vi "dfd_Set Bank Coef Infos.vi"(7 "type":T7, 8 "error in (no error)":errorcluster, 9 "gain":dbl, 10 "coefficients":dbl[](array[numeric]), 11 "bank in":T1={"mBank_Filters"=[], " mBank_#Bands"=2, "mBank_ProcMethod"=enum."General", "mBank_Coeffs"=[], "mBank_Gain"=1.0, "mBank_Type"=0} {"mBank_Type" items=["Uniform", "Non-Uniform"]; "mBank_Filters"."mMRate_SumWl" min=1 max=32 step=1; "mBank_Filters"."mMRate_InputIwl" min=1 max=32 step=1; "mBank_Filters"."mMRate_GainWl" min=1 max=32 step=1; "mBank_Filters"."mMRate_OutputWl" min=1 max=32 step=1; "mBank_Filters"."mMRate_InputWl" min=1 max=32 step=1; "mBank_Filters"."mMRate_CoefWl" min=1 max=32 step=1; "mBank_Filters"."mMRate_Mode" items=["Default"=-1, "No Rate Change"=0, "Interpolation"=1, "Decimation"=2, "Interpolated"=3, "Rational"=4]}) -> (0 "error out":errorcluster, 3 "bank out":T1={"mBank_Filters"=[], " mBank_#Bands"=2, "mBank_ProcMethod"=enum."General", "mBank_Coeffs"=[], "mBank_Gain"=1.0, "mBank_Type"=0} {"mBank_Type" items=["Uniform", "Non-Uniform"]; "mBank_Filters"."mMRate_SumWl" min=1 max=32 step=1; "mBank_Filters"."mMRate_InputIwl" min=1 max=32 step=1; "mBank_Filters"."mMRate_GainWl" min=1 max=32 step=1; "mBank_Filters"."mMRate_OutputWl" min=1 max=32 step=1; "mBank_Filters"."mMRate_InputWl" min=1 max=32 step=1; "mBank_Filters"."mMRate_CoefWl" min=1 max=32 step=1; "mBank_Filters"."mMRate_Mode" items=["Default"=-1, "No Rate Change"=0, "Interpolation"=1, "Decimation"=2, "Interpolated"=3, "Rational"=4]})   [LabVIEW 2017, in "NI_DigFilter_FilterBank.lvlib"]
uses:
  <vilib>/addons/Digital Filter Design/NI_DigFilter_FilterBank.lvlib
  <vilib>/addons/Digital Filter Design/FilterBank.llb/Object/DFD Bank Obj.ctl
  <vilib>/addons/Digital Filter Design/_Objects.llb/DFD Multirate Filter Obj.ctl
  <vilib>/addons/Digital Filter Design/_Objects.llb/DFD Multirate Mode.ctl
  <vilib>/addons/Digital Filter Design/_Objects.llb/DFD Coef Norm Type.ctl
  <vilib>/addons/Digital Filter Design/_Objects.llb/DFD Round-off Mode.ctl
  <vilib>/addons/Digital Filter Design/_Objects.llb/DFD FXP MRate Multiply Mode.ctl
  <vilib>/addons/Digital Filter Design/FilterBank.llb/Object/DFD Filter Bank Processing Method.ctl
  <vilib>/addons/Digital Filter Design/FilterBank.llb/Object/DFD Filter Bank Type.ctl
  <vilib>/addons/Digital Filter Design/_Misc.llb/dfd_Error Handlers (Single).vi
  <vilib>/addons/Digital Filter Design/NI_DigFilterLicensed.lvlib
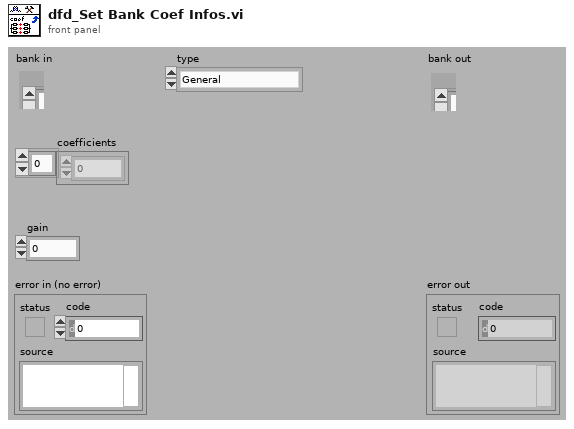
[diagram p1: front panel]
types:
  T1 = typedef "NI_DigFilter_FilterBank.lvlib/DFD Bank Obj.ctl" = cluster{"mBank_Filters":T2[], " mBank_#Bands":i32, "mBank_ProcMethod":T7, "mBank_Coeffs":dbl[], "mBank_Gain":dbl, "mBank_Type":T8}
  T2 = typedef "NI_DigFilterLicensed.lvlib/DFD Multirate Filter Obj.ctl" = cluster{"mMRate_Structure":enum16{"CIC", "FIR", "IIR", "Lattice"}, "mMRate_Mode":T3, "mMRate_Factor":i32, "mMRate_FIRParams":cluster{"mMRate_FIR_H":dbl[], "mMRate_FIR_IsNyquist?":bool, "mMRate_FIR_IsSymmetric?":bool}, "mMRate_CICParams":cluster{"mMRate_CIC_#Stage":i32, "mMRate_CIC_Lag":i32, "mMRate_CIC_Type":enum16{"Lowpass", "Highpass"}}, "mMRate_Order":i32, "mMRate_Version":string, "mMRate_Comments":string, "mMRate_RationalFactor":cluster{"mMRate_L":i32, "mMRate_M":i32}, "mMRate_Fs":dbl, "mMRate_Quantized?":bool, "mMRate_QFilterGain":dbl, "mMRate_CoefWl":i16, "mMRate_Scaling":cluster{"mMRate_ScaleByPowerOf2?":bool, "mMRate_ScaleType":T4}, "mMRate_InputWl":i16, "mMRate_OutputWl":i16, "mMRate_OutputMode":T5, "mMRate_MultMode":T6, "mMRate_BitPruning":bool, "mMRate_GainWl":i16, "mMRate_OutputFwl":i16, "mMRate_SumIwl":i16, "mMRate_InputIwl ":i16, "mMRate_SumWl":i16, "mMRate_CoefIwl":i16}
  T3 = typedef "NI_DigFilterLicensed.lvlib/DFD Multirate Mode.ctl" = i16
  T4 = typedef "NI_DigFilterLicensed.lvlib/DFD Coef Norm Type.ctl" = enum16{"No Norm", "Time Domain 1-Norm", "Time Domain 2-Norm", "Time Domain Inf-Norm"}
  T5 = typedef "NI_DigFilterLicensed.lvlib/DFD Round-off Mode.ctl" = enum16{"Nearest", "Truncation"}
  T6 = typedef "NI_DigFilterLicensed.lvlib/DFD FXP MRate Multiply Mode.ctl" = enum16{"Truncated", "Full"}
  T7 = typedef "NI_DigFilter_FilterBank.lvlib/DFD Filter Bank Processing Method.ctl" = enum16{"General", "2-Band QMF Lattice", "Cosine-Modulated"}
  T8 = typedef "NI_DigFilter_FilterBank.lvlib/DFD Filter Bank Type.ctl" = u16
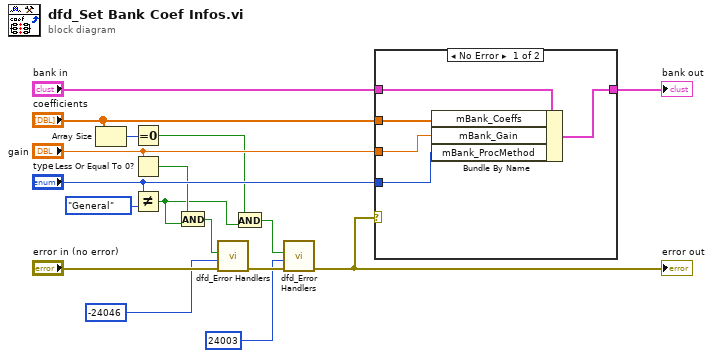
[diagram p0: block diagram]
diagram:
  n1 = Array Size(array="coefficients") -> (size(s)=w9:i32)
  n2 = Equal To 0?(x=w9) -> (x = 0?=w8:bool)
  n3 = Less Or Equal To 0?(x="gain") -> (x <= 0?=w12:bool)
  n4 = Not Equal?(x="type", y=DFD_Filter_Bank_Processing_Method."General") -> (x != y?=w11:bool)
  n5 = And(x=w12, y=w11) -> (x .and. y?=w7:bool)
  n6 = call-poly <vilib>:"dfd_Error Handlers.vi"("error in (no error)"="error in (no error)", "error code"=-24046 ("ERR_FORCED_GAIN_NOT_IN_BAND"), "condition failed?"=w7) -> ("error out"=w4:errorcluster)  [unwired: 8 in]
  n7 = And(x=w8, y=w11) -> (x .and. y?=w3:bool)
  n8 = call-poly <vilib>:"dfd_Error Handlers.vi"("error in (no error)"=w4, "error code"=24003 ("WRN_#INPUT_ZERO"), "condition failed?"=w3) -> ("error out"=w1:errorcluster)  [unwired: 8 in]
  "error out" <- w1
  n9 = case shown="No Error" w1 {
    tunnel: "type" -> [w18 _]
    tunnel: "bank in" -> [w22 w23]
    tunnel: "gain" -> [w19 _]
    tunnel: "coefficients" -> [w20 _]
    tunnel: [w21 w23] -> w16
    frame No Error {
      n10 = Bundle By Name(cluster=w22, "mBank_Coeffs"=w20, "mBank_Gain"=w19, "mBank_ProcMethod"=w18) -> (w21:T1)
    }
    frame Error {
    }
  }
  "bank out" <- w16
